vi "Dependency Migration Main.vi"(0 "library refnum":refnum<vi>, 5 "project:open":refnum<vi>, 7 "source module path":path, 11 "error in":errorcluster) -> (4 "instr containing":path[](array[path]), 15 "error out":errorcluster)   [LabVIEW 2021, in "Converter.lvlib"]
uses:
  Converter.lvlib
  Converter Reusables/Converter Reusables.lvlib
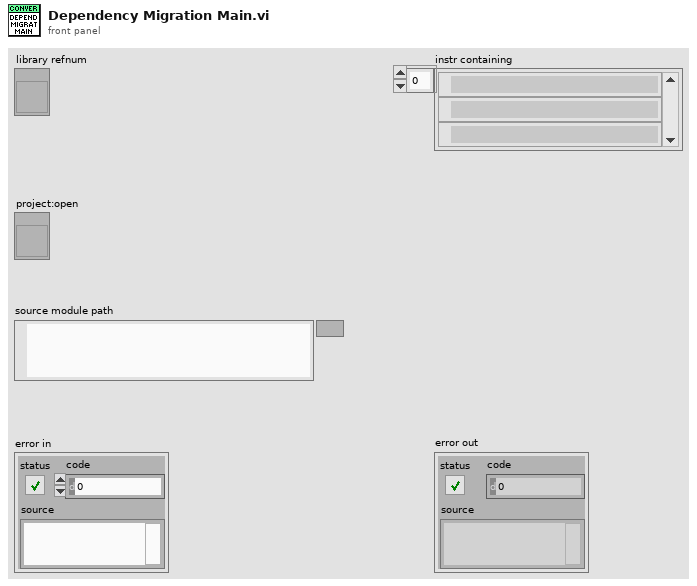
[diagram p1: front panel]
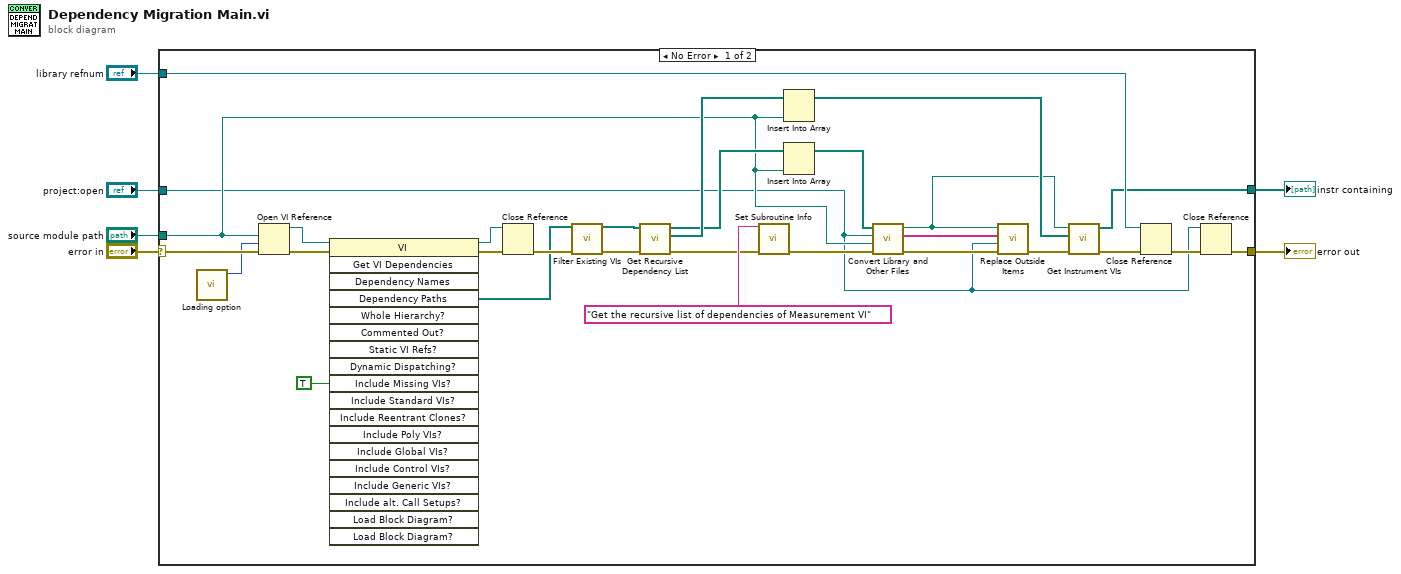
[diagram p0: block diagram]
diagram:
  n1 = case shown="No Error" "error in" {
    selector: "error in" -> [w28 w36]
    tunnel: "library refnum" -> [w31 _]
    tunnel: [w29 _] -> w5
    tunnel: [w25 w36] -> w3
    tunnel: "source module path" -> [w11 _]
    tunnel: "project:open" -> [w10 _]
    frame No Error {
      n2 = call "Loading option.vi"() -> ("options"=w19:i32)  [unwired: 11 in]
      n3 = Open VI Reference(vi path=w11, options=w19, error in (no error)=w28) -> (vi reference=w7:refnum<vi>, error out=w35:errorcluster)  [unwired: 3 in]
      n4 = invoke class="VI" method="Get VI Dependencies"(reference=w7, error in=w35, "Include Missing VIs?"=TRUE ("Include Missing Items?")) -> (reference out=w32:refnum<vi>, error out=w33:errorcluster, "Dependency Paths"=w8:path[])  [unwired: 16 in, 16 out]
      n5 = Close Reference(reference=w32, error in (no error)=w33) -> (error out=w14:errorcluster)
      n6 = call "Filter Existing VIs.vi"("dependency path"=w8, "error in"=w14) -> ("valid dep path"=w12:path[], "error out"=w13:errorcluster)  [unwired: 12 in]
      n7 = call "Get Recursive Dependency List.vi"("error in"=w13, "dependency paths"=w12) -> ("error out"=w15:errorcluster, "instr containing"=w34:path[], "array"=w16:path[])  [unwired: 7 in]
      n8 = call "Set Subroutine Info.vi"("subroutine in"="Get the recursive list of dependencies of Measurement VI" ("Subroutine In"), "error in"=w15) -> ("error out"=w18:errorcluster)  [unwired: 13 in]
      n9 = Insert Into Array(array=w34, new element=w11) -> (w30:path[])  [unwired: 1 in]
      n10 = Insert Into Array(array=w16, new element=w11) -> (w24:path[])  [unwired: 1 in]
      n11 = call "Convert Library and Other Files.vi"("error in"=w18, "main module path"=w11, "project:open"=w10, "dependency list[]"=w24) -> ("error out"=w23:errorcluster, "outside vis"=w20:string[], "destination directory"=w21:path)  [unwired: 5 in]
      n12 = call "Replace Outside Items.vi"("error in"=w23, "project:open"=w10, "outside vis"=w20, "destination directory"=w21) -> ("error out"=w22:errorcluster)  [unwired: 7 in]
      n13 = call "Get Instrument VIs.vi"("error in"=w22, "instr containing"=w30, "destination directory"=w21) -> ("error out"=w26:errorcluster, "instr containing vi[]"=w29:path[])  [unwired: 7 in]
      n14 = Close Reference(reference=w31, error in (no error)=w26) -> (error out=w27:errorcluster)
      n15 = Close Reference(reference=w10, error in (no error)=w27) -> (error out=w25:errorcluster)
    }
    frame Error {
    }
  }
  "error out" <- w3
  "instr containing" <- w5
